vi "Prototypes.vi"() -> (3 "prototypes":refnum<vi>[](array[refnum]))   [LabVIEW 2017]
uses:
  Chain1.vi
  Chain2.vi
  Chain3.vi
  Chain4.vi
  Chain5.vi
  Chain6.vi
  Normal-CSM.vi
  CSM-Testcase.lvlib
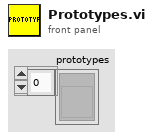
[diagram p1: front panel]
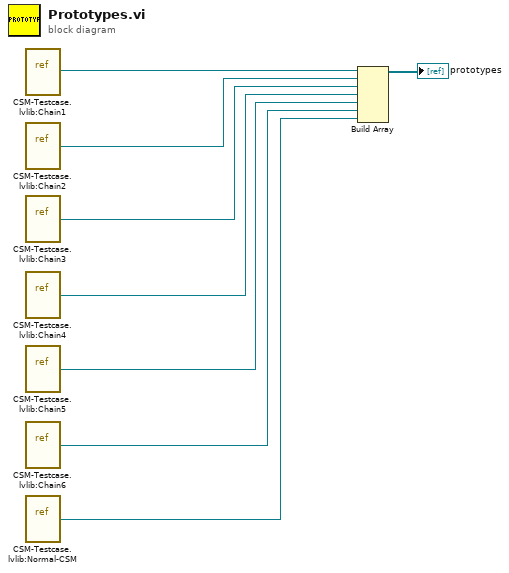
[diagram p0: block diagram]
diagram:
  n1 = vi-ref "CSM-Testcase.lvlib:Chain1.vi"() -> (w8:refnum<vi>)
  n2 = vi-ref "CSM-Testcase.lvlib:Chain2.vi"() -> (w7:refnum<vi>)
  n3 = vi-ref "CSM-Testcase.lvlib:Chain3.vi"() -> (w6:refnum<vi>)
  n4 = vi-ref "CSM-Testcase.lvlib:Chain4.vi"() -> (w5:refnum<vi>)
  n5 = vi-ref "CSM-Testcase.lvlib:Chain5.vi"() -> (w4:refnum<vi>)
  n6 = vi-ref "CSM-Testcase.lvlib:Chain6.vi"() -> (w3:refnum<vi>)
  n7 = vi-ref "CSM-Testcase.lvlib:Normal-CSM.vi"() -> (w2:refnum<vi>)
  n8 = Build Array(w8, w7, w6, w5, w4, w3, w2) -> (→"prototypes":refnum<vi>[])
